vi "Nullify.vi"(9 "Null?":bool, 10 "Number In":dbl) -> (2 "Number Out":dbl)   [LabVIEW 2015]
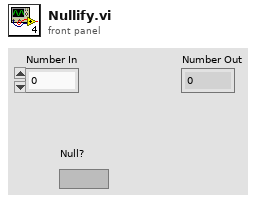
[diagram p1: front panel]
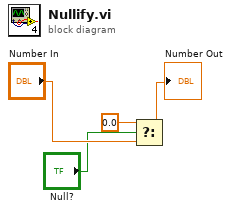
[diagram p0: block diagram]
diagram:
  n1 = Select(t=0.0, s="Null?", f="Number In") -> (s? t:f=→"Number Out":dbl)
